vi "Initial Configuration Dialog.vi"(8 "error in (no error)":errorcluster) -> (0 "error out":errorcluster, 2 "Diagnostics Basic Configuraiton":T1, 3 "Cancelled?":bool)   [LabVIEW 2015, in "Diagnostics Addon System Explorer.lvlib"]
uses:
  Diagnostics Addon System Explorer.lvlib
  Shared/Diagnostic Protocols.ctl
  Shared/CAN Interface.ctl
  Shared/Base Configuration.ctl
  Shared/Diagnostics Addon Shared.lvlib
panel:
  in  "Path":path caption="Previous Personality Path (Optional)"
  in  "Cancel":bool
  in  "OK":bool
  in  "Baud Rate":u32=250000
  in  "CAN Interface":T2
  in  "Diagnostic Protocol":T3
  in  "Database File":path caption="Database File (Optional)"
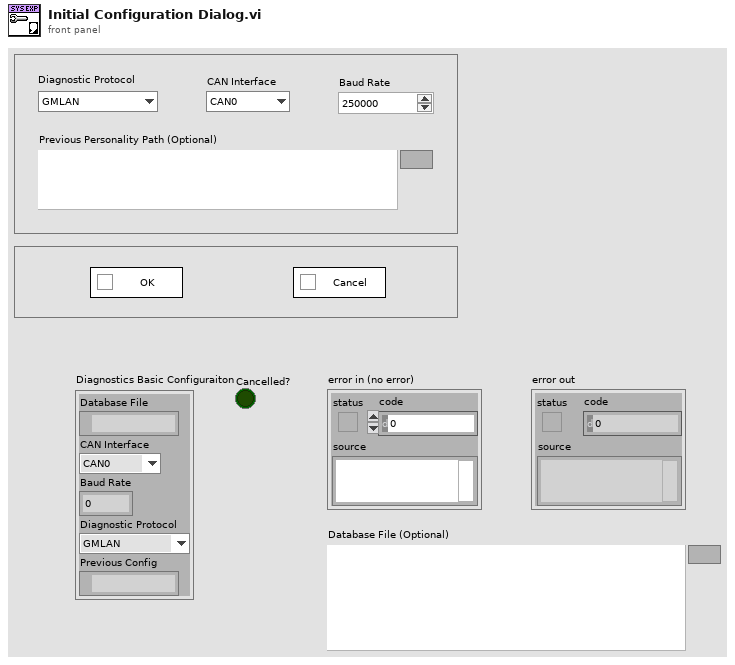
[diagram p1: front panel]
types:
  T1 = typedef "Diagnostics Addon Shared.lvlib/Base Configuration.ctl" = cluster{"Database File":path, "CAN Interface":T2, "Baud Rate":u32, "Diagnostic Protocol":T3, "Previous Config":path}
  T2 = typedef "Diagnostics Addon Shared.lvlib/CAN Interface.ctl" = enum16{"CAN0", "CAN1", "CAN2", "CAN3", "CAN4", "CAN5", "CAN6", "CAN7", "CAN8", "CAN9", "CAN10", "CAN11", "CAN12", "CAN13", "CAN14", "CAN15", "CAN16", "CAN17", "CAN18", "CAN19", "CAN20", "CAN21", "CAN22", "CAN23", "CAN24", "CAN25", "CAN26", "CAN27", "CAN28", "CAN29", "CAN30", "CAN31", "CAN32", "CAN33", "CAN34", "CAN35", "CAN36", "CAN37", "CAN38", "CAN39", "CAN40", "CAN41", "CAN42", "CAN43", "CAN44", "CAN45", "CAN46", "CAN47", "CAN48", "CAN49", "CAN50", "CAN51", "CAN52", "CAN53", "CAN54", "CAN55", "CAN56", "CAN57", "CAN58", "CAN59", "CAN60", "CAN61", "CAN62", "CAN63", "CAN 256 (Virtual)", "CAN 257 (Virtual)"}
  T3 = typedef "Diagnostics Addon Shared.lvlib/Diagnostic Protocols.ctl" = enum16{"GMLAN", "KWP-2000", "UDS"}
  T4 = enum8{"Enabled", "Disabled", "Disabled and Grayed Out"}
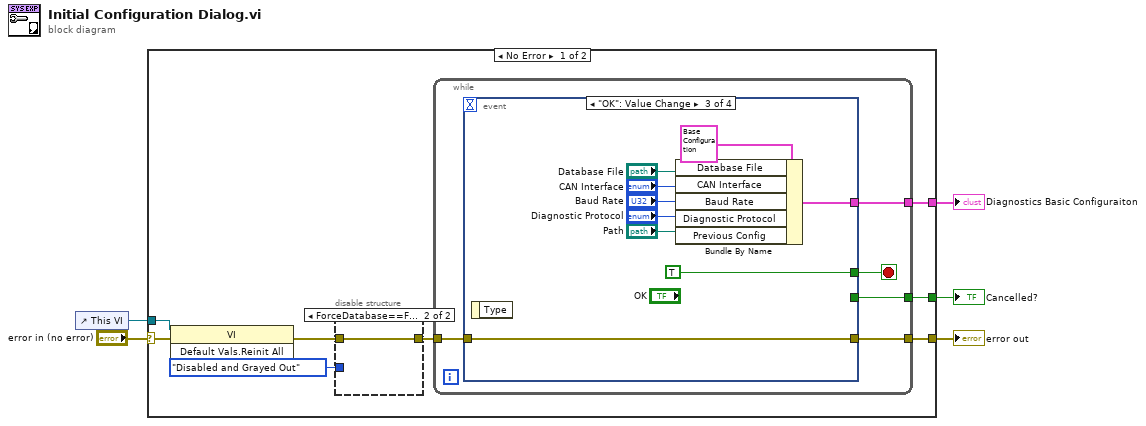
[diagram p0: block diagram]
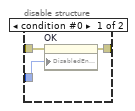
[diagram p2: hidden frame]
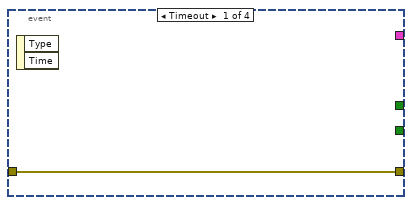
[diagram p3: hidden frame]
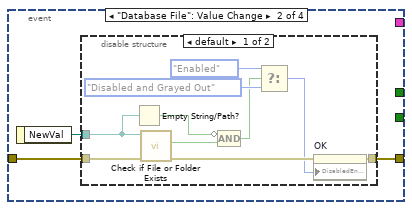
[diagram p4: hidden frame]
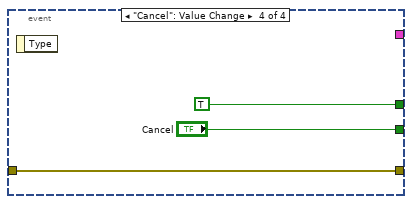
[diagram p6: hidden frame]
diagram:
  n1 = control-ref of="This VI"() -> (w1:refnum<vi>)
  n2 = case shown="No Error" "error in (no error)" {
    selector: "error in (no error)" -> [w10 w50]
    tunnel: [w13 _] -> w5
    tunnel: [w12 _] -> w4
    tunnel: [w9 w50] -> w2
    tunnel: w1 -> [w11 _]
    frame No Error {
      n3 = invoke class="VI" method="Default Vals.Reinit All"(reference=w11, error in=w10) -> (error out=w8:errorcluster)  [unwired: 1 in, 2 out]
      n4 = disable-structure shown="ForceDatabase==FALSE" {
        disable-tunnel: w8 -> [w16 w17]
        disable-tunnel: [w15 w17] -> w7
        disable-tunnel: T4."Disabled and Grayed Out" ("Disabled") -> [w14 _]
        frame condition #0 {
          n5 = property on="OK" class="Bool"(error in=w16, "DisabledEnum"=w14) -> (error out=w15:errorcluster)  [unwired: 1 in, 1 out]
        }
        frame condition #1 (active) {
        }
      }
      n6 = while {
        tunnel: [w22] -> w13
        tunnel: [w20] -> w12
        tunnel: [w18] -> w9
        tunnel: w7 -> [w19]
        stop <- w21 stop-if-true
        n7 = event shown="[2] \"OK\": Value Change" {
          selector: _ -> [_ _ _ _]
          dyn-events: _ -> [_ _ _ _]
          timeout: _ -> [_ _ _ _]
          tunnel: [_ _ _ "Cancel"] -> w22
          tunnel: [_ _ TRUE TRUE] -> w21
          tunnel: [_ _ w41 _] -> w20
          tunnel: w19 -> [w23 w25 w39 w47]
          tunnel: [w23 w26 w39 w47] -> w18
          event Timeout {
            n8 = event-data() -> ()  [unwired: 1 in, 2 out]
          }
          event "Database File": Value Change {
            n9 = event-data() -> ("NewVal"=w24:path)  [unwired: 1 in]
            n10 = disable-structure shown="default" {
              disable-tunnel: [w36 w37] -> w26
              disable-tunnel: w25 -> [w35 w37]
              disable-tunnel: w24 -> [w30 _]
              frame condition #0 {
                n11 = Empty String/Path?(string/path=w30) -> (empty?=w29:bool)
                n12 = call <vilib>:"Check if File or Folder Exists.vi"("error in (no error)"=w35, "path"=w30) -> ("error out"=w34:errorcluster, "file or folder exists?"=w28:bool)  [unwired: 7 in, 1 out]
                n13 = Compound Arithmetic op=AND(invert w29, w28) -> (w27:bool)
                n14 = Select(t=T4."Enabled" ("Disabled"), s=w27, f=T4."Disabled and Grayed Out" ("Disabled")) -> (s? t:f=w31:T4)
                n15 = property on="OK" class="Bool"(error in=w34, "DisabledEnum"=w31) -> (error out=w36:errorcluster)  [unwired: 1 in, 1 out]
              }
              frame condition #1 (active) {
              }
            }
          }
          event "OK": Value Change {
            n16 = event-data() -> ()  [unwired: 1 in, 1 out]
            n17 = Bundle By Name(cluster=T1 {"Database File"=path "", "CAN Interface"=enum."CAN0", "Baud Rate"=0, "Diagnostic Protocol"=enum."GMLAN", "Previous Config"=path ""} ("output cluster"), "Database File"="Database File", "CAN Interface"="CAN Interface", "Baud Rate"="Baud Rate", "Diagnostic Protocol"="Diagnostic Protocol", "Previous Config"="Path") -> (w41:T1)
          }
          event "Cancel": Value Change {
            n18 = event-data() -> ()  [unwired: 1 in, 1 out]
          }
        }
      }
    }
    frame Error {
    }
  }
  "Cancelled?" <- w5
  "Diagnostics Basic Configuraiton" <- w4
  "error out" <- w2
